vi "计算传输阻抗.vi"(6 "管内径[mm]":dbl, 7 "待测样品面积[mm^2]":dbl, 8 "传声器2到样品距离L[mm]":dbl, 9 "传输波数k":cdb[](array[numeric]), 10 "H21":cdb[](array[numeric]), 11 "空气特性阻抗Z0":dbl) -> (3 "传输阻抗Z":cdb[](array[numeric]))   [LabVIEW 2018]
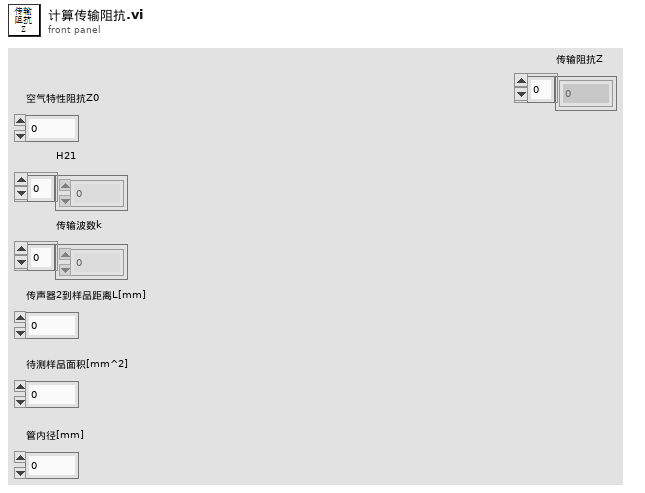
[diagram p1: front panel]
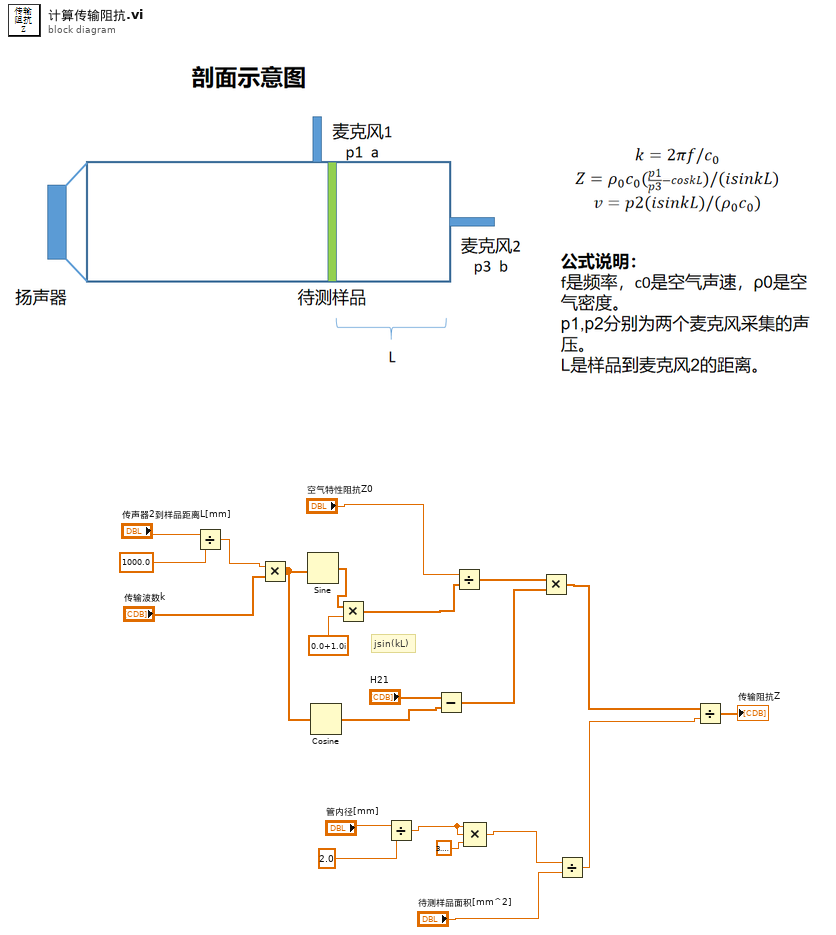
[diagram p0: block diagram]
diagram:
  # "jsin(kL)"
  n1 = Divide(x="传声器2到样品距离L[mm]", y=1000.0) -> (x/y=w18:dbl)
  n2 = Multiply(x=w18, y="传输波数k") -> (x*y=w12:cdb[])
  n3 = Sine(x=w12) -> (sin(x)=w21:cdb[])
  n4 = Cosine(x=w12) -> (cos(x)=w11:cdb[])
  n5 = Multiply(x=w21, y=cdb 0.0+1.0i) -> (x*y=w15:cdb[])
  n6 = Divide(x="管内径[mm]", y=2.0) -> (x/y=w7:dbl)
  n7 = Subtract(x="H21", y=w11) -> (x-y=w10:cdb[])
  n8 = Divide(x="空气特性阻抗Z0", y=w15) -> (x/y=w14:cdb[])
  n9 = Compound Arithmetic op=MULTIPLY(w7, w7, 3.141592653589793) -> (w5:dbl)
  n10 = Multiply(x=w14, y=w10) -> (x*y=w3:cdb[])
  n11 = Divide(x=w5, y="待测样品面积[mm^2]") -> (x/y=w2:dbl)
  n12 = Divide(x=w3, y=w2) -> (x/y=→"传输阻抗Z":cdb[])
